vi "Connection Offseted Cartesian DAO.vi"(7 "LBCB Number":T1, 8 "error in (no error)":errorcluster, 9 "CO Disp In":dbl[](array[numeric]), 10 "CO Cmd In":dbl[](array[numeric]), 11 "DAO Actions":T2) -> (0 "error out":errorcluster, 1 "CO Disp Out":dbl[](array[numeric]), 2 "CO Cmd Out":dbl[](array[numeric]))   [LabVIEW 2009]
uses:
  Data Access Objects/Metadata/DAO Actions.ctl
  Data Access Objects/Metadata/LBCB Number.ctl
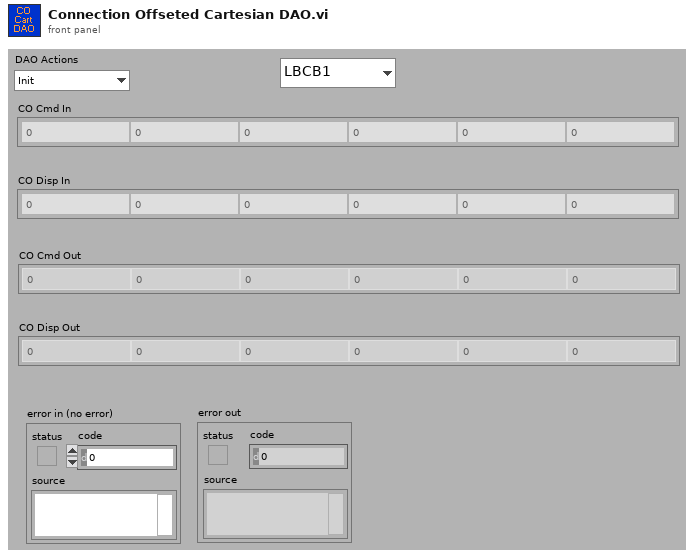
[diagram p1: front panel]
types:
  T1 = typedef "LBCB Number.ctl" = enum16{"LBCB1", "LBCB2"}
  T2 = typedef "DAO Actions.ctl" = enum16{"Init", "Get", "Set"}
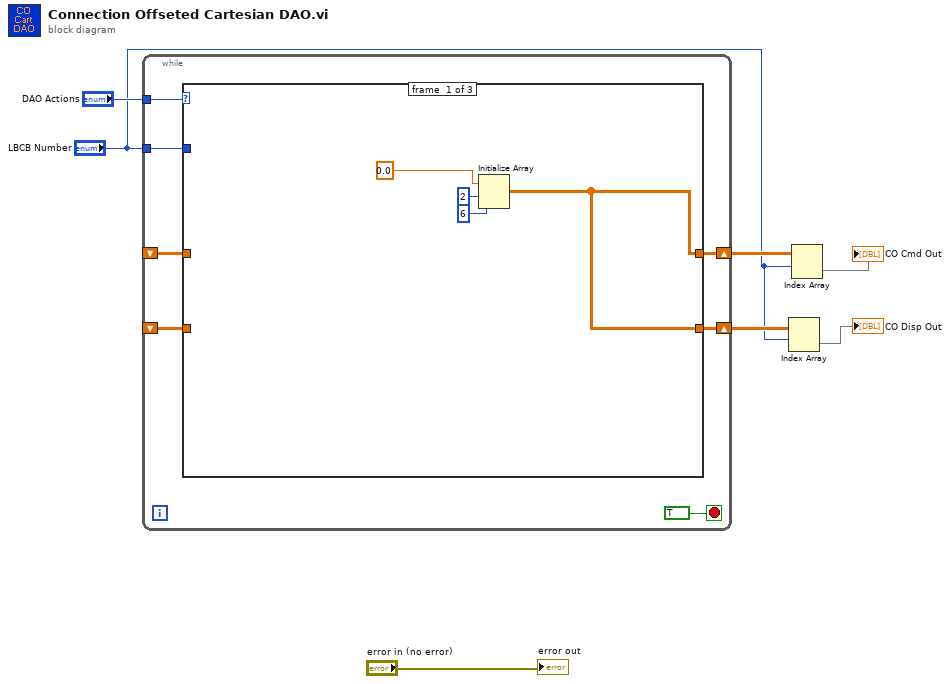
[diagram p0: block diagram]
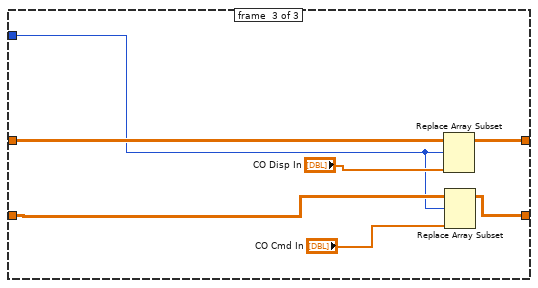
[diagram p3: hidden frame]
diagram:
  n1 = while {
    tunnel: "DAO Actions" -> [w13]
    shift-right: [w11] -> w4
    shift-left: _ -> [w9]
    shift-right: [w12] -> w5
    shift-left: _ -> [w10]
    tunnel: "LBCB Number" -> [w8]
    stop <- TRUE stop-if-true
    n2 = case shown="\"Set\"" w13 {
      tunnel: [w15 w20 w27] -> w12
      tunnel: [w15 w19 w21] -> w11
      tunnel: w10 -> [_ w20 w25]
      tunnel: w9 -> [_ w19 w24]
      tunnel: w8 -> [_ _ w22]
      frame #0 {
        n3 = Initialize Array(0.0, 2 ("dimension size"), 6 ("dimension size")) -> (w15:dbl[][])
      }
      frame #1 {
      }
      frame #2 {
        n4 = Replace Array Subset(array=w25, new element="CO Disp In", index (row)=w22) -> (w27:dbl[][])  [unwired: 1 in]
        n5 = Replace Array Subset(array=w24, new element="CO Cmd In", index (row)=w22) -> (w21:dbl[][])  [unwired: 1 in]
      }
    }
  }
  n6 = Index Array(array=w4, index (row)="LBCB Number") -> (element=→"CO Disp Out":dbl[])  [unwired: 1 in]
  n7 = Index Array(array=w5, index (row)="LBCB Number") -> (element=→"CO Cmd Out":dbl[])  [unwired: 1 in]
  "error out" <- "error in (no error)"
